vi "_jkismpp_user_lib_dir.vi"() -> (0 "<LabVIEW>":path, 1 "jkismpp_user.lib_dir":path)   [LabVIEW 2014]
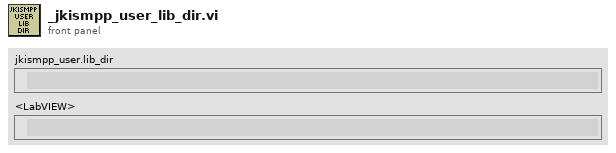
[diagram p1: front panel]
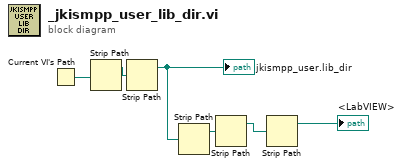
[diagram p0: block diagram]
diagram:
  n1 = Current VI's Path() -> (path=w6:path)
  n2 = Strip Path(path=w6) -> (stripped path=w5:path)  [unwired: 1 out]
  n3 = Strip Path(path=w5) -> (stripped path=w3:path)  [unwired: 1 out]
  "jkismpp_user.lib_dir" <- w3
  n4 = Strip Path(path=w3) -> (stripped path=w4:path)  [unwired: 1 out]
  n5 = Strip Path(path=w4) -> (stripped path=w2:path)  [unwired: 1 out]
  n6 = Strip Path(path=w2) -> (stripped path=→"<LabVIEW>":path)  [unwired: 1 out]
